vi "RichToFlatnixnet_grpc_DbOpenDatabaseResponse.vi"(5 "OutputClusterType":T1, 11 "InputCluster":T3) -> (3 "OutputCluster":T1)   [LabVIEW 2025, in "xnet-grpc_client.lvlib"]
uses:
  nixnet_grpc_DbOpenDatabaseResponse.ctl
  nidevice_grpc_Session.ctl
  nixnet_grpc_DbOpenDatabaseResponse_Flat.ctl
  nidevice_grpc_Session_Flat.ctl
  xnet-grpc_client.lvlib
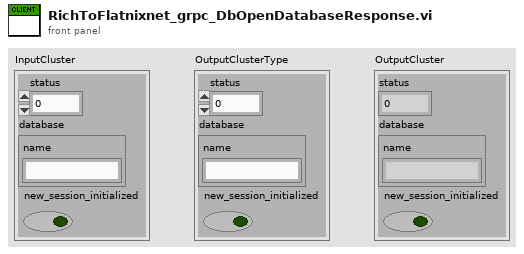
[diagram p1: front panel]
types:
  T1 = typedef "xnet-grpc_client.lvlib/nixnet_grpc_DbOpenDatabaseResponse_Flat.ctl" = cluster{"status":i32, "database":T2, "new_session_initialized":bool}
  T2 = typedef "xnet-grpc_client.lvlib/nidevice_grpc_Session_Flat.ctl" = cluster{"name":string}
  T3 = typedef "xnet-grpc_client.lvlib/nixnet_grpc_DbOpenDatabaseResponse.ctl" = cluster{"status":i32, "database":T4, "new_session_initialized":bool}
  T4 = typedef "xnet-grpc_client.lvlib/nidevice_grpc_Session.ctl" = cluster{"name":string}
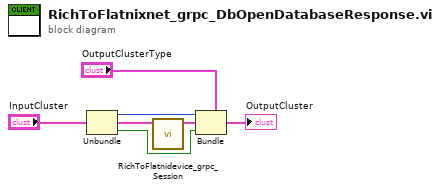
[diagram p0: block diagram]
diagram:
  n1 = Unbundle "Unbundle"("InputCluster") -> ("status"=w4:i32, "database"=w3:T4, "new_session_initialized"=w1:bool)
  n2 = call "RichToFlatnidevice_grpc_Session.vi"("InputCluster"=w3) -> ("OutputCluster"=w2:T2)  [unwired: 10 in]
  n3 = Bundle "Bundle"(cluster="OutputClusterType", "status"=w4, "database"=w2, "new_session_initialized"=w1) -> (→"OutputCluster":T1)
